vi "Day02-04_SubVI2.vi"(8 "더하기 4":dbl, 9 "빼기 3":dbl, 10 "더하기 2":dbl, 11 "더하기1":dbl) -> (2 "출력결과":dbl)   [LabVIEW 2021]
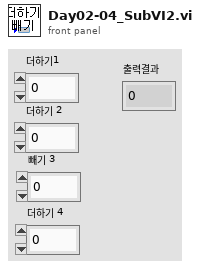
[diagram p1: front panel]
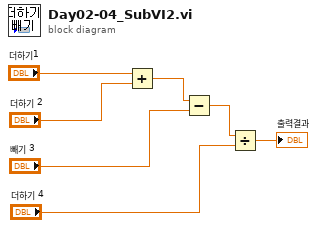
[diagram p0: block diagram]
diagram:
  n1 = Add(x="더하기1", y="더하기 2") -> (x+y=w5:dbl)
  n2 = Subtract(x=w5, y="빼기 3") -> (x-y=w2:dbl)
  n3 = Divide(x=w2, y="더하기 4") -> (x/y=→"출력결과":dbl)
